vi "my.vi"() -> ()   [LabVIEW 2011]
panel:
  out "appended array":dbl[][](array[numeric])
  out "ln(x)":dbl
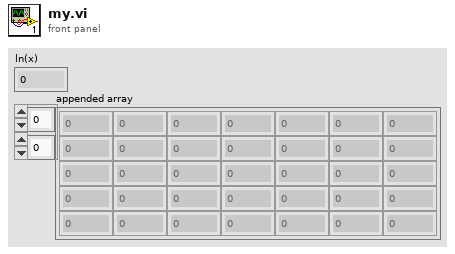
[diagram p1: front panel]
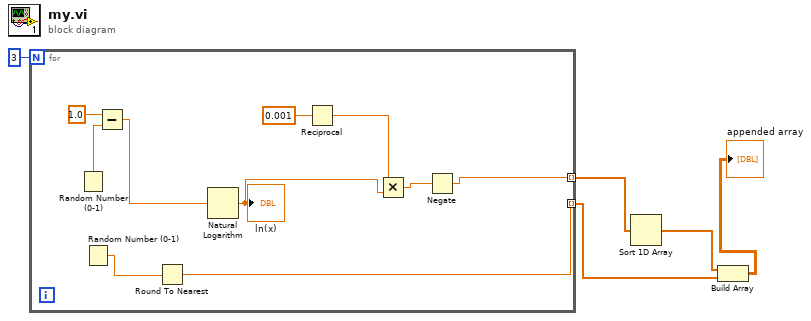
[diagram p0: block diagram]
diagram:
  n1 = for {
    N: 3 -> [_]
    tunnel: [w8] -> w4 mode=indexing
    tunnel: [w6] -> w3 mode=indexing
    n2 = Random Number (0-1)() -> (number: 0 to 1=w15:dbl)
    n3 = Random Number (0-1)() -> (number: 0 to 1=w7:dbl)
    n4 = Subtract(x=1.0, y=w15) -> (x-y=w13:dbl)
    n5 = Round To Nearest(number=w7) -> (nearest integer value=w6:dbl)
    n6 = Natural Logarithm(1:w13) -> (0:w12:dbl)
    "ln(x)" <- w12
    n7 = Reciprocal(x=0.001) -> (1/x=w11:dbl)
    n8 = Multiply(x=w11, y=w12) -> (x*y=w9:dbl)
    n9 = Negate(x=w9) -> (-x=w8:dbl)
  }
  n10 = Sort 1D Array(array=w4) -> (sorted array=w2:dbl[])
  n11 = Build Array(w2, w3) -> (→"appended array":dbl[][])
